vi "Initialize.vi"(8 "error in":errorcluster, 10 "resource":string, 11 "host in":refnum<class "LIA Debugging.lvclass">) -> (0 "error out":errorcluster, 3 "host out":refnum<class "LIA Debugging.lvclass">)   [LabVIEW 2018, in "LIA Debugging.lvclass"]
uses:
  LIA Debugging.lvclass
  C:/Users/jfernand/Repositories/Lock-In-Amplifier/Shared/lib/interface/Interface FPGA/LIA Host Interface FPGA.lvclass
  Shared/lib/interface/Interface FPGA/Public/Session Data.ctl
  Shared/lib/interface/Interface FPGA/LIA Host Interface FPGA.lvclass/LIA Host Interface FPGA.ctl
  <vilib>/FPGAPlugInAG/PXIe-7976R/niLvFpga_Open_PXIe-7976R.vi
  <vilib>/rvi/interface/common/dynamic/niFpgaDynamicAddResources.vi
  <vilib>/Utility/error.llb/Error Cluster From Error Code.vi
  <vilib>/rvi/errors/niLvFpgaAdjustHostInterfaceError.vi
  <vilib>/rvi/interface/nirviOpenFPGA/nirviOpenFPGA.xnode
  FPGA Bitfiles/LIA Debugging FPGA.lvbitx
  <vilib>/rvi/interface/nirviReadWriteControl/nirviReadWriteControl.xnode
  Shared/lib/host/Lock-In Amplifier Example Host.lvlib
  Shared/lib/interface/Interface FPGA/LIA Host Interface FPGA.lvclass
  NiFpgaLv.dll
  <vilib>/rvi/interface/Simulation/niFpgaSimulationCallBeginRW.vi
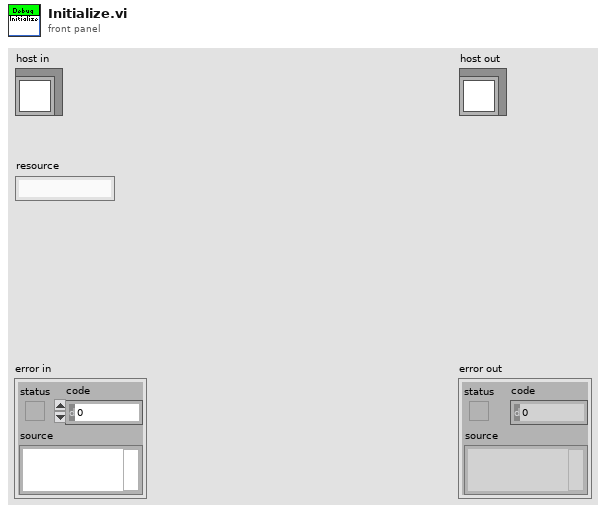
[diagram p1: front panel]
types:
  T1 = typedef "LIA Host Interface FPGA.lvclass/Session Data.ctl" = cluster{"fpga session":refnum<k20>, "record length":u32[]}
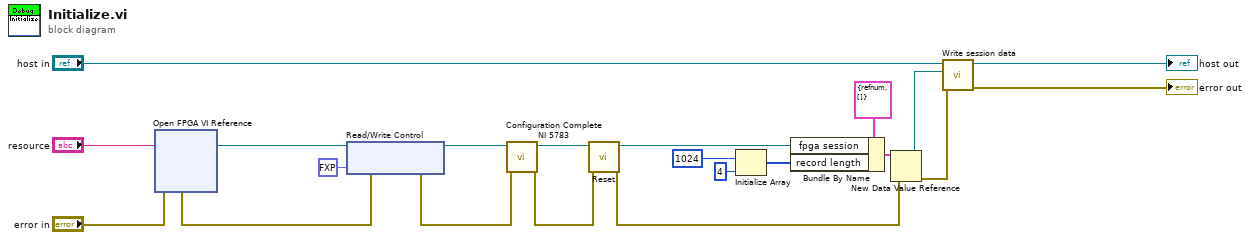
[diagram p0: block diagram]
diagram:
  n1 = xnode "Open FPGA VI Reference"("error in"="error in", "resource name"="resource") -> ("FPGA VI Reference Out"=w17:refnum<k20>, "error out"=w13:errorcluster)
  n2 = xnode "Read/Write Control"("FPGA VI Reference In"=w17, "error in"=w13, "ao.noise gain 3"=fxp<+,18,1> 0.0) -> ("FPGA VI Reference Out"=w14:refnum<k20>, "error out"=w12:errorcluster)
  n3 = call "Configuration Complete NI 5783.vi"("error in"=w12, "fpga session in"=w14) -> ("error out"=w16:errorcluster, "fpga session out"=w15:refnum<k20>)  [unwired: 7 in, 1 out]
  n4 = call "Reset.vi"("error in"=w16, "fpga session in"=w15) -> ("error out"=w18:errorcluster, "fpga session out"=w21:refnum<k20>)  [unwired: 8 in]
  n5 = Initialize Array(u32 1024 ("element"), 4 ("dimension size")) -> (w8:u32[])
  n6 = Bundle By Name(cluster=T1 {"fpga session"=refnum, "record length"=[]} ("session data"), "fpga session"=w21, "record length"=w8) -> (w19:T1)
  n7 = New Data Value Reference(data value=w19, error in=w18) -> (data value reference=w4:refnum<data-value>, error out=w3:errorcluster)
  n8 = call "Write session data.vi"("error in (no error)"=w3, "session data"=w4, "LIA Host Interface FPGA in"="host in") -> ("error out"=→"error out":errorcluster, "LIA Host Interface FPGA out"=→"host out":refnum<class "LIA Debugging.lvclass">)  [unwired: 7 in]
